vi "Calculate Phase.vi"(8 "error in (no error)":errorcluster, 9 "reset phase":bool, 10 "phase out":dbl[](array[numeric]), 11 "config phase":dbl[](array[numeric])) -> (0 "error out":errorcluster, 1 "reset?":bool, 3 "adjusted phase":dbl[](array[numeric]))   [LabVIEW 2019, in "Generator.lvclass"]
uses:
  Generator.lvclass
  Program Files (x86)/National Instruments/LabVIEW 2020/user.lib/_OpenG.lib/array/array.llb/Empty 1D Array (DBL)__ogtk.vi
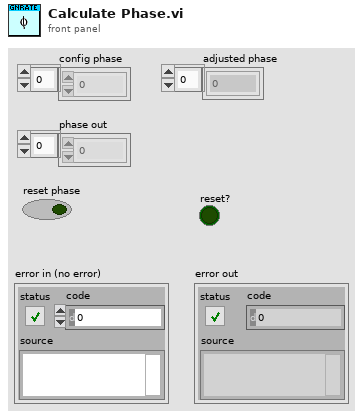
[diagram p1: front panel]
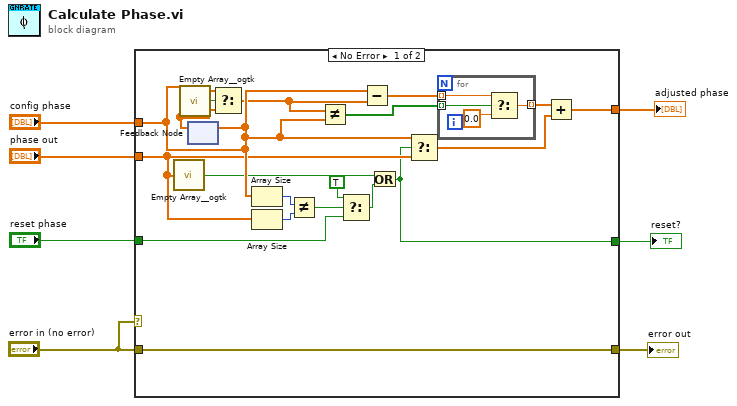
[diagram p0: block diagram]
diagram:
  n1 = case shown="No Error" "error in (no error)" {
    tunnel: "reset phase" -> [w26 w31]
    tunnel: "config phase" -> [w25 w32]
    tunnel: "phase out" -> [w17 _]
    tunnel: [w15 w32] -> w4
    tunnel: [w9 w33] -> w3
    tunnel: "error in (no error)" -> [w9 w33]
    tunnel: [w8 w31] -> w1
    frame No Error {
      n2 = call-poly "Empty Array__ogtk.vi"("Array"=w17) -> ("Empty Array?"=w10:bool)  [unwired: 8 in]
      n3 = feedback #1() -> (w12:dbl[])  [unwired: 1 in]
      n4 = call-poly "Empty Array__ogtk.vi"("Array"=w12) -> ("Empty Array?"=w11:bool)  [unwired: 8 in]
      n5 = feedback-in #1(w25) -> ()
      n6 = Select(t=w25, s=w11, f=w12) -> (s? t:f=w13:dbl[])
      n7 = Array Size(array=w25) -> (size(s)=w16:i32)
      n8 = Array Size(array=w17) -> (size(s)=w24:i32)
      n9 = Not Equal?(x=w16, y=w24) -> (x != y?=w18:bool)
      n10 = Not Equal?(x=w13, y=w25) -> (x != y?=w22:bool[])
      n11 = Select(t=TRUE, s=w18, f=w26) -> (s? t:f=w19:bool)
      n12 = Subtract(x=w25, y=w13) -> (x-y=w14:dbl[])
      n13 = Or(x=w10, y=w19) -> (x .or. y?=w8:bool)
      n14 = Select(t=w25, s=w8, f=w17) -> (s? t:f=w23:dbl[])
      n15 = for {
        tunnel: w22 -> [w30] mode=indexing
        tunnel: w14 -> [w29] mode=indexing
        tunnel: [w27] -> w21 mode=indexing
        n16 = Select(t=w29, s=w30, f=0.0) -> (s? t:f=w27:dbl)
      }
      n17 = Add(x=w21, y=w23) -> (x+y=w15:dbl[])
    }
    frame Error {
    }
  }
  "adjusted phase" <- w4
  "error out" <- w3
  "reset?" <- w1
